vi "Open Gyro.vi"(9 "Analog Channel":T1) -> ()   [LabVIEW 2013]
uses:
  <vilib>/Rock Robotics/SystemInterfaces/AI/FPGA_AIChannel.ctl
  Gyro Global.vi
panel:
  in  "Gyro ID (1 or 2)":i32
  in  "Gain":dbl=0.07
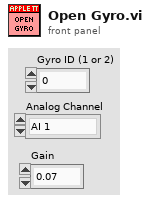
[diagram p1: front panel]
types:
  T1 = typedef "FPGA_AIChannel.ctl" = enum8{"AI 1", "AI 2", "AI 3", "AI 4", "AI 5", "AI 6", "AI 7", "AI 8", "Invalid"}
  T2 = typedef "WPI_AnalogChannelDevRef.ctl" = cluster{"DevStatus":errorcluster, "Analog Module":T3, "Analog Channel":T1}
  T3 = typedef "FPGA_TypedefAnalogModule.ctl" = enum16{"Analog Module 1", "Analog Module 2"}
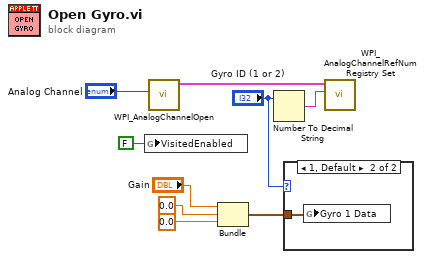
[diagram p0: block diagram]
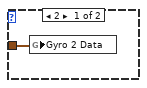
[diagram p2: hidden frame]
diagram:
  n1 = global write "Gyro Global.vi" "VisitedEnabled"(FALSE ("VisitedEnabled")) -> ()
  n2 = call <vilib>:"WPI_AnalogChannelOpen.vi"("Analog Channel"="Analog Channel") -> ("AIDeviceRef"=w8:T2)  [unwired: 9 in, 1 out]
  n3 = Bundle("Gain"="Gain", 0.0, 0.0) -> (w1:cluster{"Gain":dbl, dbl, dbl})  [unwired: 1 in]
  n4 = Number To Decimal String(number="Gyro ID (1 or 2)") -> (decimal integer string=w6:string)  [unwired: 1 in]
  n5 = case shown="1, Default" "Gyro ID (1 or 2)" {
    tunnel: w1 -> [w10 w11]
    frame 2 {
      n6 = global write "Gyro Global.vi" "Gyro 2 Data"(w10) -> ()
    }
    frame 1, Default {
      n7 = global write "Gyro Global.vi" "Gyro 1 Data"(w11) -> ()
    }
  }
  n8 = call <vilib>:"WPI_AnalogChannelRefNum Registry Set.vi"("refnum name"=w6, "AIDeviceRef"=w8) -> ()  [unwired: 8 in, 2 out]
